vi "6.vi"() -> ()   [LabVIEW 2022 SP3]
panel:
  in  "Numeric":dbl
  out "GREEN":bool
  out "YELLOW":bool
  out "RED":bool
  # "Aditya Singh\n     2315005"
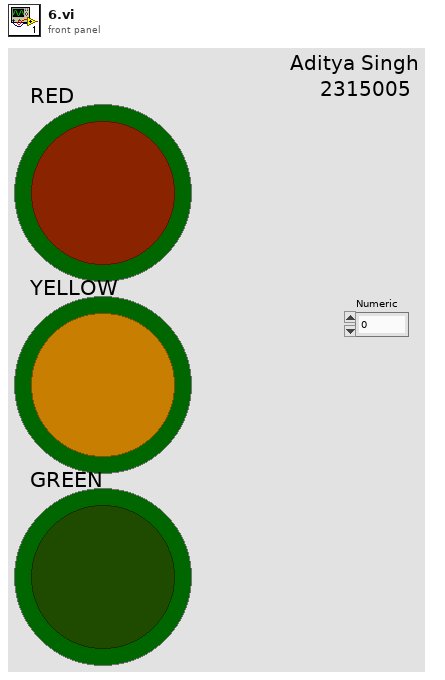
[diagram p1: front panel]
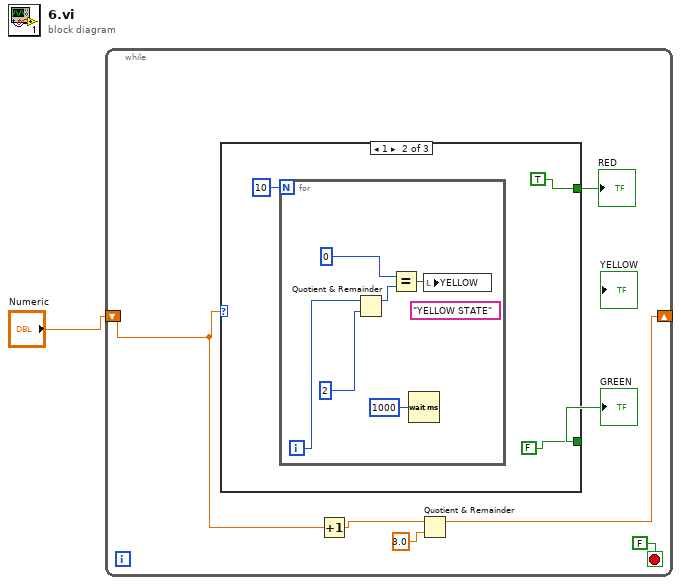
[diagram p0: block diagram]
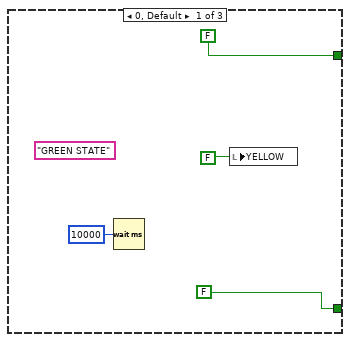
[diagram p2: hidden frame]
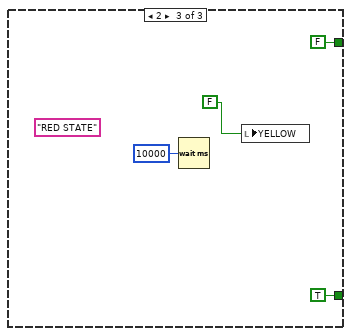
[diagram p3: hidden frame]
diagram:
  n1 = while {
    shift-right: [w4] -> _
    shift-left: "Numeric" -> [w7]
    stop <- FALSE ("stop") stop-if-true
    n2 = case shown="1" w7 {
      tunnel: [FALSE FALSE TRUE] -> w3
      tunnel: [FALSE TRUE FALSE] -> w2
      frame 0, Default {
        (unwired) "GREEN STATE"
        n3 = Wait (ms)(milliseconds to wait=u32 10000) -> ()  [unwired: 1 out]
        n4 = local write "YELLOW"(FALSE) -> ()
      }
      frame 1 {
        n5 = for {
          N: 10 -> [_]
          i -> [w21]
          (unwired) "YELLOW STATE"
          n6 = Quotient & Remainder(x=w21, y=2) -> (x-y*floor(x/y)=w20:i32)  [unwired: 1 out]
          n7 = Equal?(x=0, y=w20) -> (x = y?=w17:bool)
          n8 = Wait (ms)(milliseconds to wait=u32 1000) -> ()  [unwired: 1 out]
          n9 = local write "YELLOW"(w17) -> ()
        }
      }
      frame 2 {
        (unwired) "RED STATE"
        n10 = Wait (ms)(milliseconds to wait=u32 10000) -> ()  [unwired: 1 out]
        n11 = local write "YELLOW"(FALSE) -> ()
      }
    }
    "RED" <- w2
    "GREEN" <- w3
    n12 = Increment(x=w7) -> (x+1=w6:dbl)
    n13 = Quotient & Remainder(x=w6, y=3.0) -> (x-y*floor(x/y)=w4:dbl)  [unwired: 1 out]
  }
